vi "Moving Average Method 2.vi"() -> ()   [LabVIEW 2019]
panel:
  out "Array":dbl[](array[numeric])
  in  "Sensor":dbl(slide) min=-1.0 max=1.0 scale=-1.0..1.0
  out "Plot":cluster{dbl, dbl}(graph)
  in  "Stop":bool
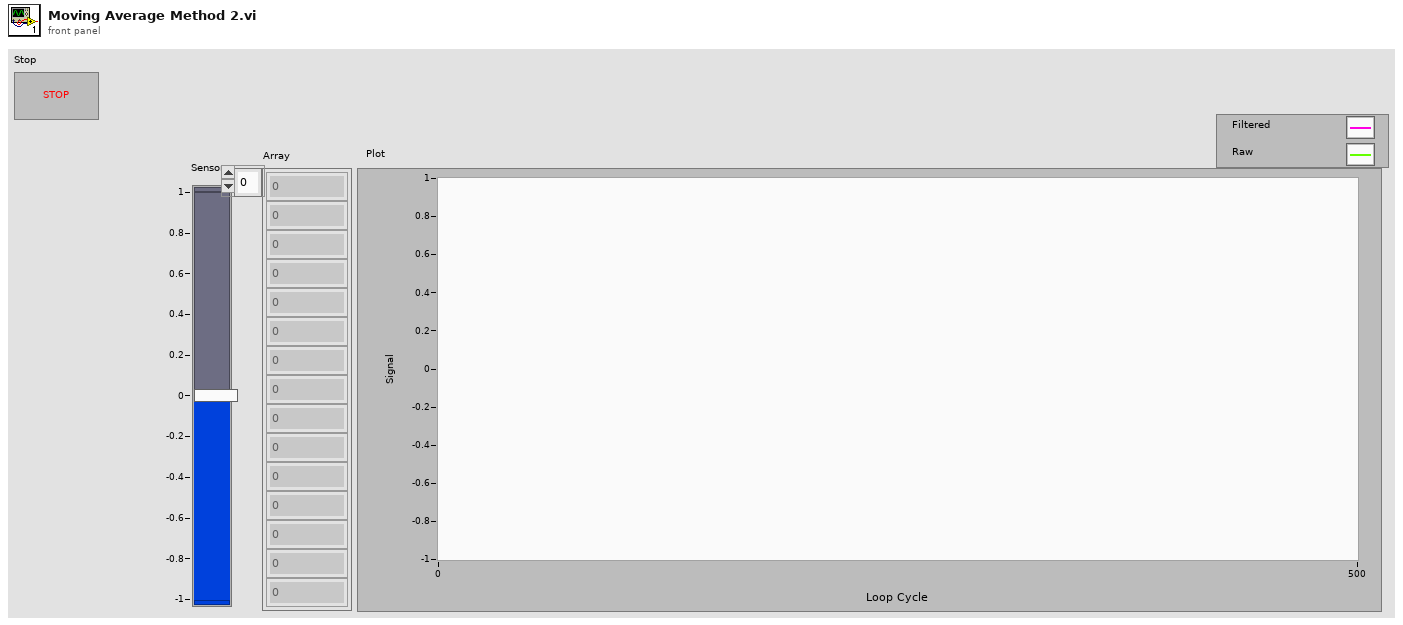
[diagram p1: front panel]
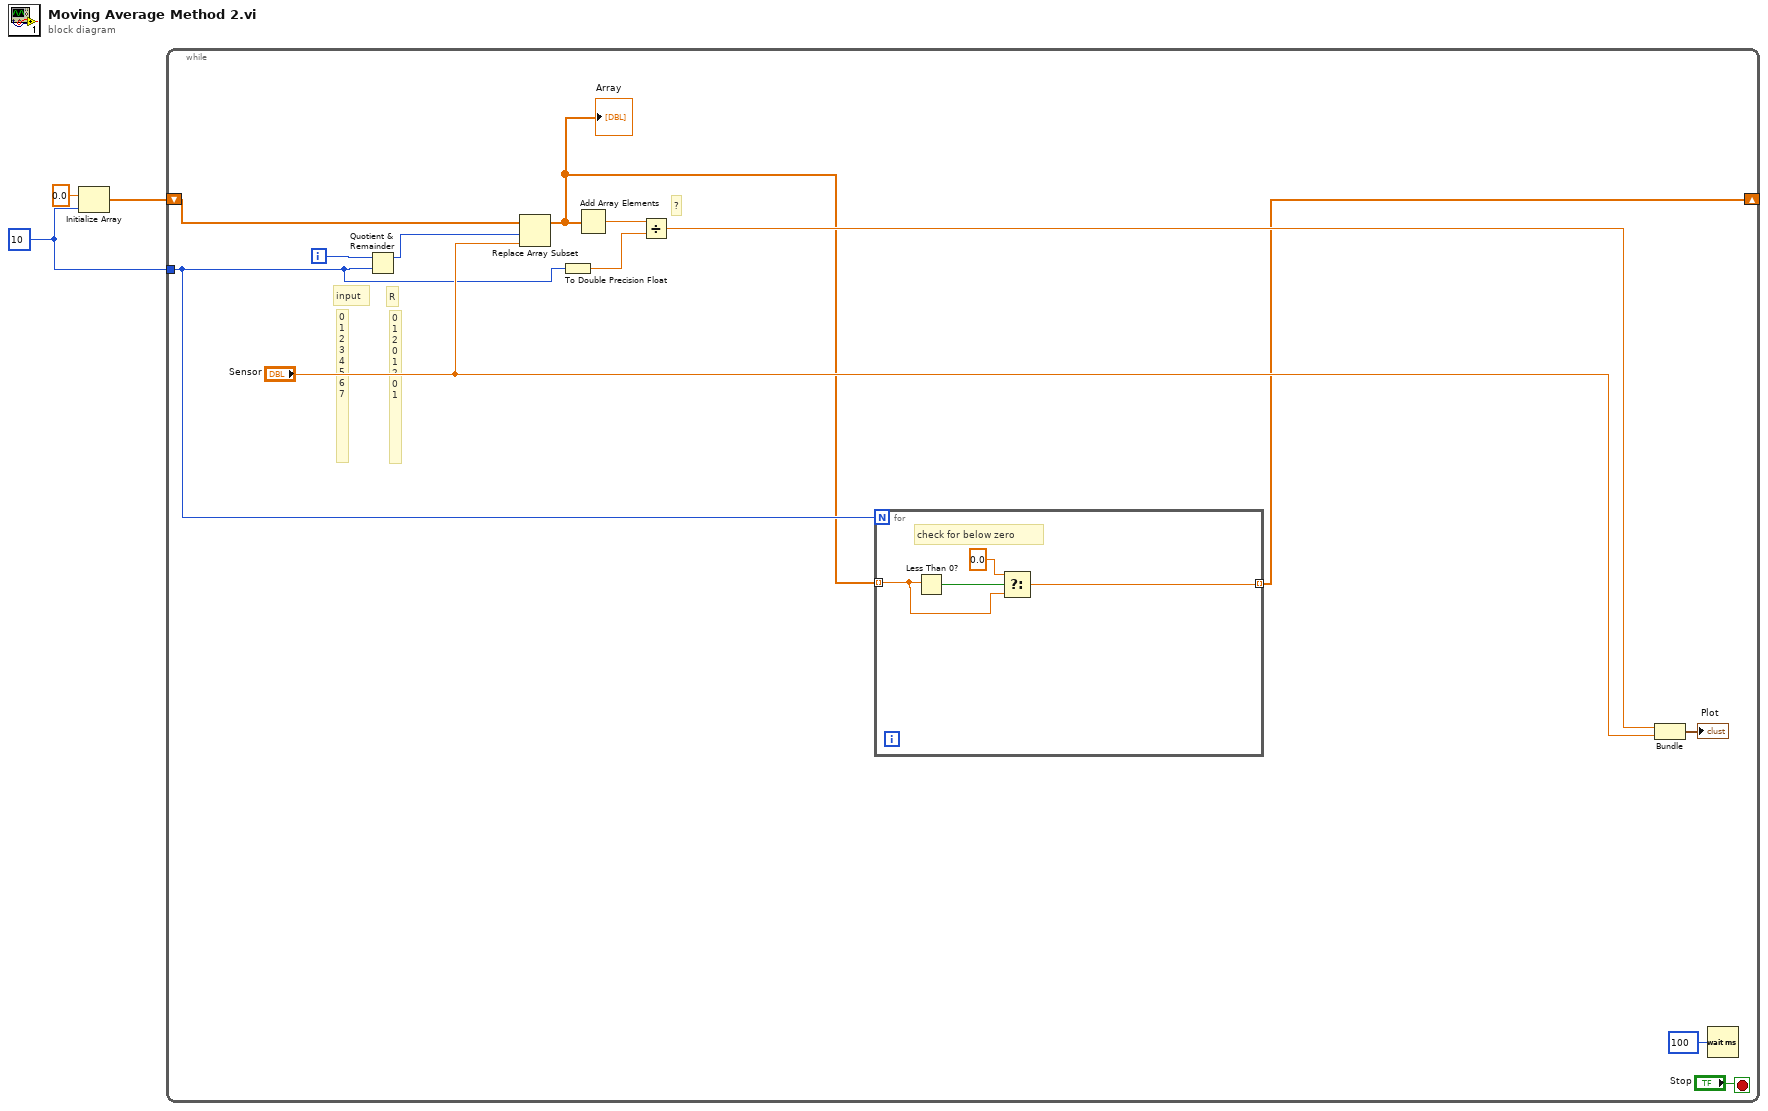
[diagram p0: block diagram]
diagram:
  w1 = 10 ("dimension size")
  n1 = Initialize Array(0.0 ("element"), w1) -> (w2:dbl[])
  n2 = while {
    tunnel: w1 -> [w6]
    shift-right: [w4] -> _
    shift-left: w2 -> [w10]
    i -> [w13]
    stop <- "Stop" stop-if-true
    # "?"
    # "R"
    # "0\n1\n2\n0\n1\n2\n0\n1"
    # "input"
    # "0\n1\n2\n3\n4\n5\n6\n7"
    n3 = Quotient & Remainder(x=w13, y=w6) -> (x-y*floor(x/y)=w12:i32)  [unwired: 1 out]
    n4 = Replace Array Subset(array=w10, new element="Sensor", index=w12) -> (w5:dbl[])
    "Array" <- w5
    n5 = To Double Precision Float(number=w6) -> (double precision float=w8:dbl)
    n6 = Add Array Elements(numeric array=w5) -> (sum=w9:dbl)
    n7 = Divide(x=w9, y=w8) -> (x/y=w7:dbl)
    n8 = for {
      N: w6 -> [_]
      tunnel: w5 -> [w19] mode=indexing
      tunnel: [w17] -> w4 mode=indexing
      # "check for below zero"
      n9 = Less Than 0?(x=w19) -> (x < 0?=w20:bool)
      n10 = Select(t=0.0, s=w20, f=w19) -> (s? t:f=w17:dbl)
    }
    n11 = Bundle(w7, "Sensor"="Sensor") -> (→"Plot":cluster{dbl, "Sensor":dbl})  [unwired: 1 in]
    n12 = Wait (ms)(milliseconds to wait=u32 100) -> ()  [unwired: 1 out]
  }
